vi "Do.vi"(8 "error in (no error)":errorcluster, 10 "Actor in":refnum<class "Actor.lvclass">, 11 "AIO Actor Msg":refnum<class "AIO Actor Msg.lvclass">) -> (0 "error out":errorcluster, 2 "Actor out":refnum<class "Actor.lvclass">)   [LabVIEW 2024, in "AIO Actor.lvlib" / "AIO Actor Msg.lvclass"]
doc: "(<B>Filename</B>: Actor Framework.lvlib:Message.lvclass:Do.vi)\n\nDefines what a message does when it is received by an actor. Generally, a message instructs an actor to invoke one of its methods. By default, this method does nothing. A child class must override it to define behavior. Create a child class by using the Actor Framework Message Maker dialog box."
uses:
  AIO Actor Msg.lvclass
  <vilib>/ActorFramework/Actor/Actor.lvclass
  Actor/AIO.lvclass
  C:/Program Files (x86)/National Instruments/LabVIEW 2024/vi.lib/ActorFramework/Actor/Actor.lvclass
  AIO Actor Msg.lvclass/AIO Actor Msg.ctl
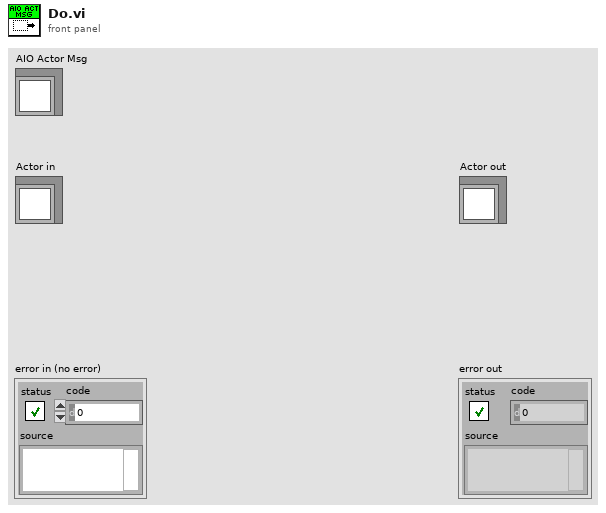
[diagram p1: front panel]
types:
  T1 = typedef "AO Type.ctl" = enum16{"Static", "Streaming", "StopStreaming"}
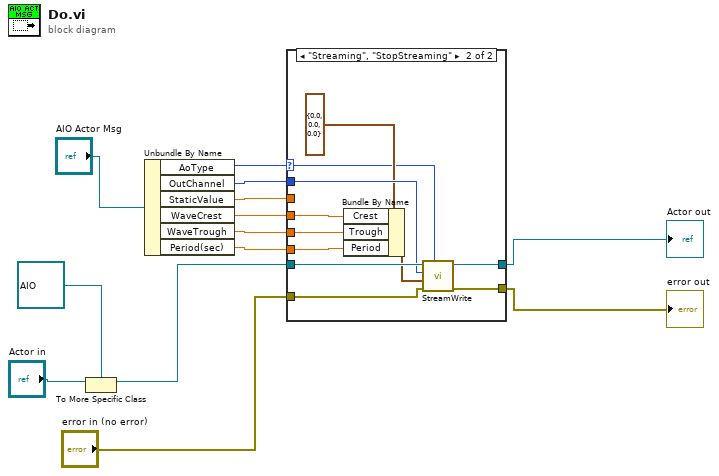
[diagram p0: block diagram]
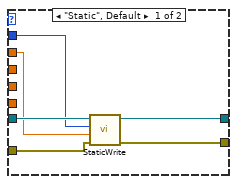
[diagram p2: hidden frame]
diagram:
  n1 = To More Specific Class(target class=refnum<class "AIO.lvclass"> refnum ("AIO Actor.lvlib:AIO.lvclass"), reference="Actor in") -> (specific class reference=w9:refnum<class "AIO.lvclass">)  [unwired: 1 in, 1 out]
  n2 = Unbundle By Name("AIO Actor Msg") -> ("AoType"=w10:T1, "OutChannel"=w8:u8, "StaticValue"=w7:dbl, "WaveCrest"=w3:dbl, "WaveTrough"=w2:dbl, "Period(sec)"=w1:dbl)
  n3 = case shown="\"Streaming\", \"StopStreaming\"" w10 {
    selector: w10 -> [_ w20]
    tunnel: w9 -> [w19 w30]
    tunnel: w8 -> [w18 w29]
    tunnel: w7 -> [w17 _]
    tunnel: "error in (no error)" -> [w16 w28]
    tunnel: [w15 w21] -> w4
    tunnel: [w14 w22] -> w5
    tunnel: w3 -> [_ w26]
    tunnel: w2 -> [_ w25]
    tunnel: w1 -> [_ w24]
    frame "Static", Default {
      n4 = call "StaticWrite.vi"("error in (no error)"=w16, "StaticValue"=w17, "Channel"=w18, "AIO in"=w19) -> ("error out"=w15:errorcluster, "AIO out"=w14:refnum<class "AIO.lvclass">)  [unwired: 6 in]
    }
    frame "Streaming", "StopStreaming" {
      n5 = Bundle By Name(cluster=cluster{"Crest":dbl, "Trough":dbl, "Period":dbl} {"Crest"=0.0, "Trough"=0.0, "Period"=0.0} ("WavePara"), "Crest"=w26, "Trough"=w25, "Period"=w24) -> (w23:cluster{"Crest":dbl, "Trough":dbl, "Period":dbl})
      n6 = call "StreamWrite.vi"("AoType"=w20, "error in (no error)"=w28, "WavePara"=w23, "Channel"=w29, "AIO in"=w30) -> ("error out"=w21:errorcluster, "AIO out"=w22:refnum<class "AIO.lvclass">)  [unwired: 5 in]
    }
  }
  "error out" <- w4
  "Actor out" <- w5
